vi "Continuous Serial Write and Read2.vi"() -> ()   [LabVIEW 2015]
doc: "本范例根据用户指示，对串口执行读写操作。范例运行时可按下“写入”或“读取”按钮，以及修改“读数”。\n\n设置的串口参数必须匹配连接仪器或设备的参数。本范例中，“读数”参数可指定串口读取的字节数。如端口字节超过指定的字节数，超出部分将不会被读取。如端口字节数少于指定的字节数，将返回超时错误。\n\n本范例可扩展流控制选项以包括XON和XOFF，从而允许用户选择控制字符。同时，用户可启用或禁用中止符。部分设备需要通过终止符确定命令字符串的结束位置。部分设备将发送终止符以说明待读取数据的末端。本范例演示了缓冲区中检测到终止符时，结束“读取”操作或添加终止符至“写入”数据末端的方法。"
uses:
  H:/Program Files (x86)/National Instruments/LabVIEW 2015/examples/Instrument IO/Serial/support/Serial - Settings.ctl
  H:/Program Files (x86)/National Instruments/LabVIEW 2015/examples/Instrument IO/Serial/support/Serial - XON-XOFF Characters.ctl
  H:/Program Files (x86)/National Instruments/LabVIEW 2015/examples/Instrument IO/Serial/support/Serial - ASCII Characters.ctl
  <vilib>/Instr/_visa.llb/VISA Configure Serial Port (Instr).vi
  <userlib>/add/add.lvlib
panel:
  in  "镜像转90":bool=TRUE
  out "Z标尺.刻度值[] 2":cluster{"数值输入控件":dbl, "颜色盒":u32}[](array[cluster])=[{"数值输入控件"=0.0, "颜色盒"=11929}, {"数值输入控件"=5.0, "颜色盒"=16860}, {"数值输入控件"=10.0, "颜色盒"=7303167}, {"数值输入控件"=15.0, "颜色盒"=655113}, {"数值输入控件"=20.0, "颜色盒"=8716164}, {"数值输入控件"=25.0, "颜色盒"=16750634}, {"数值输入控件"=30.0, "颜色盒"=16726329}, {"数值输入控件"=35.0, "颜色盒"=14876672}]
  in  "温度补偿":dbl=5.0
  in  "milliseconds to wait":u32=5
  in  "插值":bool=TRUE
  in  "显示范围":u16=24
  in  "Z标尺.刻度值[]":cluster{"数值输入控件":dbl, "颜色盒":u32}[](array[cluster])=[{"数值输入控件"=0.0, "颜色盒"=11929}, {"数值输入控件"=5.0, "颜色盒"=16860}, {"数值输入控件"=10.0, "颜色盒"=7303167}, {"数值输入控件"=15.0, "颜色盒"=655113}, {"数值输入控件"=20.0, "颜色盒"=8716164}, {"数值输入控件"=25.0, "颜色盒"=16750634}, {"数值输入控件"=30.0, "颜色盒"=16726329}, {"数值输入控件"=35.0, "颜色盒"=14876672}]
  in  "插值率":dbl=3.0
  out "子字符串之后":string
  out "强度图":dbl[][](graph)
  in  "终止符":u8=10 format="%.0x"
  in  "终止符时结束写入？":bool=TRUE
  in  "停止":bool
  in  "命令":string="*IDN?"
  in  "读数":u32=1000
  out "响应":string
  in  "写入":bool
  in  "读取":bool=TRUE
  in  "XON/XOFF字符":T1={"XON"=enum."DC1", "XOFF"=enum."DC3"}
  in  "串口设置":T3={"波特率"=115200, "数据比特"=8, "奇偶"=enum."None", "停止位"=10, "流控制"=0} {"流控制" items=["无"=0, "XON/XOFF"=1, "RTS/CTS"=2, "DTR/DSR"=4]; "停止位" items=["1.0"=10, "1.5"=15, "2.0"=20]; "数据比特" min=5 max=8 step=1; "波特率" items=["75"=75, "110"=110, "134"=134, "150"=150, "300"=300, "600"=600, "1200"=1200, "1800"=1800, "2400"=2400, "4800"=4800, "7200"=7200, "9600"=9600, "14400"=14400, "19200"=19200, "28800"=28800, "38400"=38400, "56000"=56000, "57600"=57600, "115200"=115200, "128000"=128000, "230400"=230400]}
  in  "终止符时结束读取？":bool=TRUE
  in  "VISA资源名称":refnum<visa-resource-name>="COM4"
  # "概述：演示在循环中使用VISA函数连续写入命令至串口仪器或从串口仪器读取响应。\n要求：NI-VISA驱动程序\n操作步骤：\n1. 运行VI。\n2. 指定命令并单击写入按钮。\n3. 单击读取按钮读取响应。\n4. 单击停止按钮停止VI。"
  # "0xA相当于'\\n'字符，为换行符。"
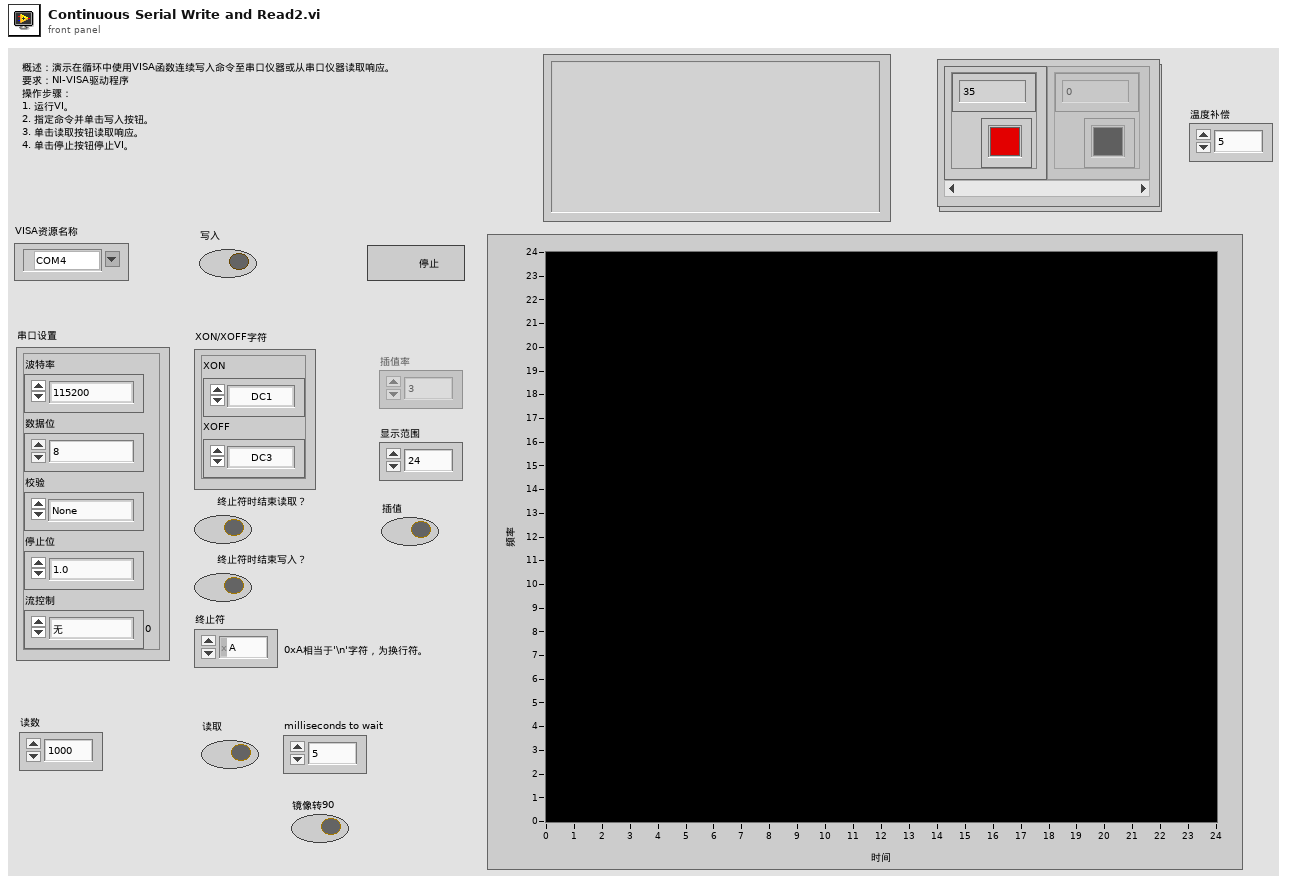
[diagram p1: front panel]
types:
  T1 = typedef "Serial - XON-XOFF Characters.ctl" = cluster{"XON":T2, "XOFF":T2}
  T2 = typedef "Serial - ASCII Characters.ctl" = enum16{"NUL", "SOH", "STX", "ETX", "EOT", "ENQ", "ACK", "BEL", "BS", "HT", "LF", "VT", "FF", "CR", "SO", "SI", "DLE", "DC1", "DC2", "DC3", "DC4", "NAK", "SYN", "ETB", "CAN", "EM", "SUB", "ESC", "FS", "GS", "RS", "US", "SP", "!", "\"", "#", "$", "%", "&", "'", "(", ")", "*", "+", ",", "- (-)", ".", "/", "0", "1", "2", "3", "4", "5", "6", "7", "8", "9", ":", ";", "<", "=", ">", "?", "@", "A", "B", "C", "D", "E", "F", "G", "H", "I", "J", "K", "L", "M", "N", "O", "P", "Q", "R", "S", "T", "U", "V", "W", "X", "Y", "Z", "[", "\\", "]", "^", "_", "`", "a", "b", "c", "d", "e", "f", "g", "h", "i", "j", "k", "l", "m", "n", "o", "p", "q", "r", "s", "t", "u", "v", "w", "x", "y", "z", "{", "|", "}", "~"}
  T3 = typedef "Serial - Settings.ctl" = cluster{"波特率":u32, "数据比特":u16, "奇偶":enum16{"None", "Odd", "Even", "Mark", "Space"}, "停止位":u16, "流控制":u16}
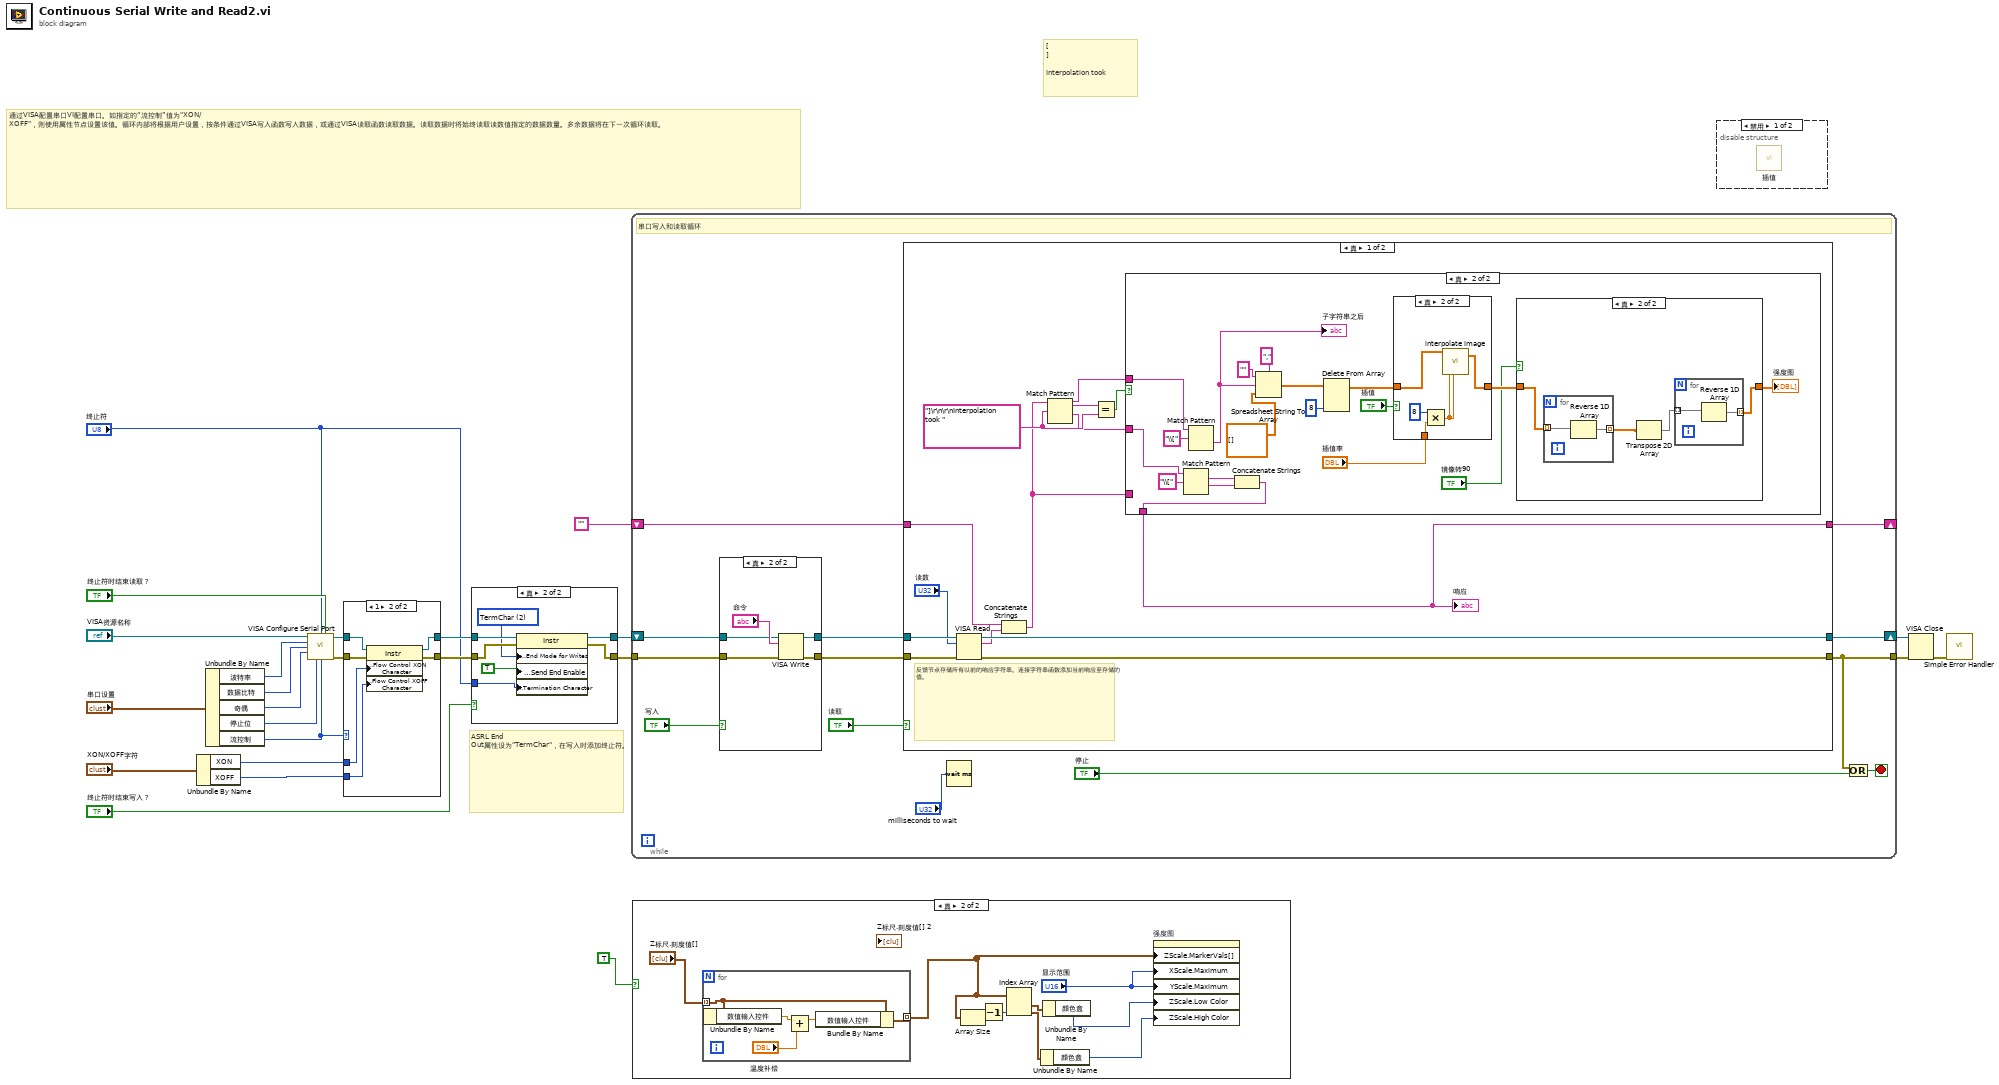
[diagram p0: block diagram]
diagram:
  # "[\n]\n\nInterpolation took"
  # "ASRL End Out属性设为\"TermChar\"，在写入时添加终止符。"
  # "通过VISA配置串口VI配置串口。如指定的“流控制”值为\"XON/XOFF\"，则使用属性节点设置该值。循环内部将根据用户设置，按条件通过VISA写入函数写入数据，或通过VISA读取函数读取数据。读取数据时将始终读取读数值指定的数据数量。多余数据将在下一次循环读取。"
  n1 = Unbundle By Name("XON/XOFF字符") -> ("XON"=w10:T2, "XOFF"=w9:T2)
  n2 = Unbundle By Name("串口设置") -> ("波特率"=w17:u32, "数据比特"=w18:u16, "奇偶"=w19:enum16{"None", "Odd", "Even", "Mark", "Space"}, "停止位"=w20:u16, "流控制"=w11:u16)
  n3 = call-poly "VISA Configure Serial Port"("VISA resource name"="VISA资源名称", "termination char\n(0xA = '\\n' = LF)"="终止符", "Enable Termination\nChar (T)"="终止符时结束读取？", "baud rate (9600)"=w17, "data bits (8)"=w18, "parity (0:none)"=w19, "stop bits (10: 1 bit)"=w20, "flow control (0:none)"=w11) -> ("VISA resource name out"=w21:refnum<visa-resource-name>, "error out"=w22:errorcluster)  [unwired: 2 in, 4 out]
  n4 = case shown="1" w11 {
    tunnel: [w25 w32] -> w8
    tunnel: [w26 w31] -> w6
    tunnel: w22 -> [w25 w30]
    tunnel: w21 -> [w26 w29]
    tunnel: w10 -> [_ w28]
    tunnel: w9 -> [_ w27]
    frame Default {
    }
    frame 1 {
      n5 = property class="Instr"(reference=w29, error in=w30, "Serial Settings:Flow Control XON Character"=w28, "Serial Settings:Flow Control XOFF Character"=w27) -> (reference out=w31:refnum<visa-resource-name>, error out=w32:errorcluster)
    }
  }
  n6 = case shown="真" "终止符时结束写入？" {
    tunnel: w6 -> [w33 w41]
    tunnel: w8 -> [w34 w40]
    tunnel: [w33 w39] -> w5
    tunnel: [w34 w38] -> w7
    tunnel: "终止符" -> [_ w36]
    frame False {
    }
    frame True {
      w37 = u16 2 items=["None", "LastBit", "TermChar", "Break"] ("Serial Settings:Serial End Mode for Writes")
      n7 = property class="Instr"(reference=w41, error in=w40, "Serial Settings:End Mode for Writes"=w37, "Message Based Settings:Send End Enable"=TRUE, "Message Based Settings:Termination Character"=w36) -> (reference out=w39:refnum<visa-resource-name>, error out=w38:errorcluster)
    }
  }
  n8 = while {
    shift-right: [w54] -> w12
    shift-left: w5 -> [w53]
    tunnel: w7 -> [w52]
    tunnel: [w46] -> w13
    shift-right: [w42] -> _
    shift-left: "" -> [w43]
    stop <- w47 stop-if-true
    # "串口写入和读取循环"
    n9 = case shown="真" "写入" {
      tunnel: w53 -> [w56 w60]
      tunnel: w52 -> [w55 w59]
      tunnel: [w56 w58] -> w51
      tunnel: [w55 w57] -> w50
      frame False {
      }
      frame True {
        n10 = VISA Write(VISA resource name=w60, write buffer="命令", error in (no error)=w59) -> (VISA resource name out=w58:refnum<visa-resource-name>, error out=w57:errorcluster)  [unwired: 1 out]
      }
    }
    n11 = case shown="真" "读取" {
      tunnel: [w73 w112] -> w54
      tunnel: w51 -> [w75 w112]
      tunnel: [w71 w111] -> w46
      tunnel: w50 -> [w74 w111]
      tunnel: w43 -> [w64 _]
      tunnel: [w63 _] -> w42
      frame True {
        w69 = "]\r\n\r\nInterpolation took "
        # "反馈节点存储所有以前的响应字符串。连接字符串函数添加当前响应至存储的值。"
        n12 = VISA Read(VISA resource name=w75, byte count="读数", error in (no error)=w74) -> (VISA resource name out=w73:refnum<visa-resource-name>, read buffer=w70:string, error out=w71:errorcluster)  [unwired: 1 out]
        n13 = Concatenate Strings(w64, w70) -> (w66:string)
        n14 = Match Pattern(string=w66, regular expression=w69) -> (before substring=w62:string, match substring=w65:string, after substring=w67:string)  [unwired: 1 in, 1 out]
        n15 = Equal?(x=w65, y=w69) -> (x = y?=w68:bool)
        n16 = case shown="真" w68 {
          tunnel: w67 -> [_ w92]
          tunnel: [w76 w89] -> w63
          tunnel: w66 -> [w76 _]
          tunnel: w62 -> [_ w94]
          frame False {
          }
          frame True {
            n17 = Match Pattern(string=w92, regular expression="\\[") -> (match substring=w91:string, after substring=w90:string)  [unwired: 1 in, 2 out]
            n18 = Match Pattern(string=w94, regular expression="\\[") -> (after substring=w88:string)  [unwired: 1 in, 3 out]
            "子字符串之后" <- w88
            n19 = Concatenate Strings(w91, w90) -> (w89:string)
            n20 = Spreadsheet String To Array(delimiter (Tab)="," ("分隔符(Tab)"), format string="" ("分隔符(Tab)"), spreadsheet string=w88, array type (2D Dbl)=dbl[][] []) -> (array=w85:dbl[][])
            n21 = Delete From Array(array=w85, index (col)=8 ("禁用的索引 (列)")) -> (array with subset deleted=w82:dbl[][])  [unwired: 2 in, 1 out]
            n22 = case shown="真" "插值" {
              tunnel: w82 -> [w105 w110]
              tunnel: [w105 w109] -> w81
              tunnel: "插值率" -> [_ w107]
              frame False {
              }
              frame True {
                n23 = Multiply(x=8, y=w107) -> (x*y=w106:dbl)
                n24 = call <userlib>:"interpolate image.vi"("src"=w110, "dest_rows"=w106, "dest_cols"=w106) -> ("dest out"=w109:sgl[][])  [unwired: 14 in, 2 out]
              }
            }
            n25 = case shown="真" "镜像转90" {
              tunnel: w81 -> [w96 w100]
              tunnel: [w96 w97] -> w78
              frame False {
              }
              frame True {
                n26 = for {
                  tunnel: w100 -> [w104] mode=indexing
                  tunnel: [w103] -> w99 mode=indexing
                  n27 = Reverse 1D Array(array=w104) -> (reversed array=w103:dbl[])
                }
                n28 = Transpose 2D Array(2D array=w99) -> (transposed array=w98:dbl[][])
                n29 = for {
                  tunnel: w98 -> [w102] mode=indexing
                  tunnel: [w101] -> w97 mode=indexing
                  n30 = Reverse 1D Array(array=w102) -> (reversed array=w101:dbl[])
                }
              }
            }
            "强度图" <- w78
          }
        }
        "响应" <- w63
      }
      frame False {
      }
    }
    n31 = Wait (ms)(milliseconds to wait="milliseconds to wait") -> ()  [unwired: 1 out]
    n32 = Or(x=w46, y="停止") -> (x .or. y?=w47:bool)
  }
  n33 = case shown="真" TRUE ("更新") {
    frame False {
    }
    frame True {
      n34 = for {
        tunnel: "Z标尺.刻度值[]" -> [w126] mode=indexing
        tunnel: [w122] -> w113 mode=indexing
        n35 = Unbundle By Name(w126) -> ("数值输入控件"=w125:dbl)
        n36 = Add(x=w125, y="温度补偿") -> (x+y=w124:dbl)
        n37 = Bundle By Name(cluster=w126, "数值输入控件"=w124) -> (w122:cluster{"数值输入控件":dbl, "颜色盒":u32})
      }
      n38 = Array Size(array=w113) -> (size(s)=w118:i32)
      n39 = Decrement(x=w118) -> (x-1=w117:i32)
      n40 = Index Array(array=w113, index #2=w117) -> (element #1=w120:cluster{"数值输入控件":dbl, "颜色盒":u32}, element #2=w116:cluster{"数值输入控件":dbl, "颜色盒":u32})  [unwired: 1 in]
      n41 = Unbundle By Name(w116) -> ("颜色盒"=w115:u32)
      n42 = Unbundle By Name(w120) -> ("颜色盒"=w119:u32)
      n43 = property on="强度图" class="强度图 (严格)"("ZScale.MarkerVals[]"=w113, "XScale.Maximum"="显示范围", "YScale.Maximum"="显示范围", "ZScale.Low Color"=w119, "ZScale.High Color"=w115) -> ()  [unwired: 2 in, 2 out]
    }
  }
  n44 = disable-structure shown="禁用" {
    frame Disabled {
      n45 = call "插值.vi"() -> ()  [unwired: 10 in, 2 out]
    }
    frame Enabled {
    }
  }
  n46 = VISA Close(VISA resource name=w12, error in (no error)=w13) -> (error out=w14:errorcluster)
  n47 = call <vilib>:"Simple Error Handler.vi"("error in (no error)"=w14) -> ()  [unwired: 1 in, 8 out]
